vi "Generate SPI Command Frame.vi"(9 "Address":u16 format="%.0x", 11 "R/W":enum16{"Write", "Read"}(ring)=enum."Read") -> (3 "SPI Command Frame":bool[](array[boolean]))   [LabVIEW 2023]
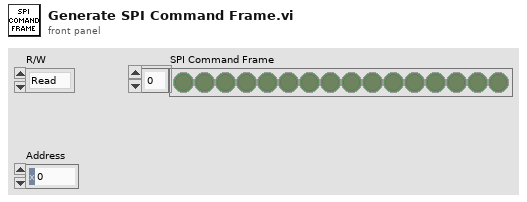
[diagram p1: front panel]
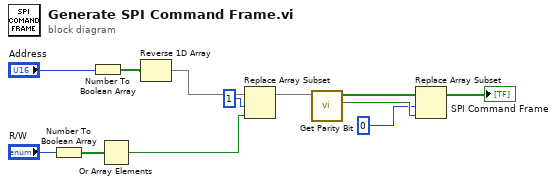
[diagram p0: block diagram]
diagram:
  n1 = Number To Boolean Array(number="R/W") -> (Boolean array=w8:bool[])
  n2 = Number To Boolean Array(number="Address") -> (Boolean array=w11:bool[])
  n3 = Or Array Elements(Boolean array=w8) -> (logical OR=w6:bool)
  n4 = Reverse 1D Array(array=w11) -> (reversed array=w10:bool[])
  n5 = Replace Array Subset(array=w10, new element=w6, index=1) -> (w5:bool[])
  n6 = call "Get Parity Bit.vi"("Array in"=w5) -> ("Parity Bit"=w3:bool, "Array out"=w4:bool[])  [unwired: 9 in]
  n7 = Replace Array Subset(array=w4, new element=w3, index=0) -> (→"SPI Command Frame":bool[])
